vi "Send_Data.vi"(0 "Poss":dbl) -> (1 "value":dbl, 2 "error out":errorcluster)   [LabVIEW 2017]
uses:
  <vilib>/myRIO/Instrument Drivers/Onboard IO/AI Block/typedefs/AI Block Reference.ctl
  <vilib>/myRIO/Common/Instrument Driver Framework/Utilities/typedefs/myRIO Generic Hardware Reference.ctl
  <vilib>/myRIO/Common/Instrument Driver Framework/Utilities/typedefs/Hardware Version Enum.ctl
  <vilib>/myRIO/Common/Instrument Driver Framework/Utilities/typedefs/myRIO v1.0 Reference.ctl
  <vilib>/myRIO/Common/Instrument Driver Framework/Utilities/typedefs/Generic FPGA Reference.ctl
  <vilib>/myRIO/Common/Instrument Driver Framework/myRIO v1.0/AI Block/typedefs/AI Block Channels List.ctl
  <vilib>/myRIO/Common/Instrument Driver Framework/myRIO v1.0/AI Block/typedefs/AI Block Channels Enum.ctl
  <vilib>/myRIO/Common/Instrument Driver Framework/Utilities/typedefs/Analog Scaling Constants.ctl
  <vilib>/userdefined/High Color/nirio_resource_hc.ctl
  <vilib>/myRIO/Common/Instrument Driver Framework/Utilities/vis/Is FPGA Ref Available.vi
  <vilib>/myRIO/Common/Instrument Driver Framework/myRIO v1.0/AI Block/vis/myRIO v1.1 Open Throughput AI (N Samples).vi
  <vilib>/myRIO/Instrument Drivers/Onboard IO/AI Block/vis/Read.vi
  <vilib>/myRIO/Common/Instrument Driver Framework/Utilities/vis/Validate Channels.vi
  <vilib>/Utility/VariantDataType/GetNumericInfo.vi
  <vilib>/Utility/error.llb/Error Cluster From Error Code.vi
  <vilib>/myRIO/Common/Instrument Driver Framework/myRIO v1.0/myRIO v1.1 Open Throughput.vi
  <vilib>/myRIO/Common/Instrument Driver Framework/myRIO v1.0/AI Block/vis/myRIO v1.0 Get Scaling Constants AI Block.vi
  <vilib>/myRIO/Common/Instrument Driver Framework/myRIO v1.0/AI Block/vis/myRIO v1.0 Reserve AI Block.vi
  <vilib>/myRIO/Common/Instrument Driver Framework/myRIO v1.0/myRIO v1.0 Close.vi
  <vilib>/myRIO/Common/Instrument Driver Framework/myRIO v1.0/AI Block/vis/myRIO v1.0 AI Block Read.vi
  <vilib>/myRIO/Express VI/Onboard IO/AI/AI Express VI.xnode
  <vilib>/myRIO/Instrument Drivers/Onboard IO/AI Block/vis/myRIO AI N Samples Open.xnode
  <vilib>/myRIO/Instrument Drivers/Onboard IO/AI Block/AI Block.lvlib
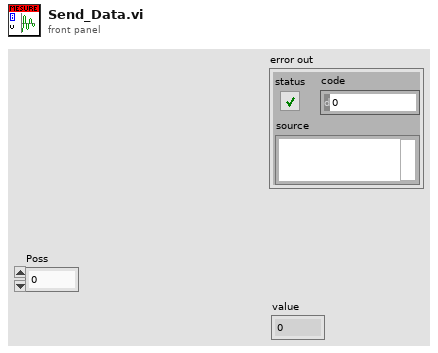
[diagram p1: front panel]
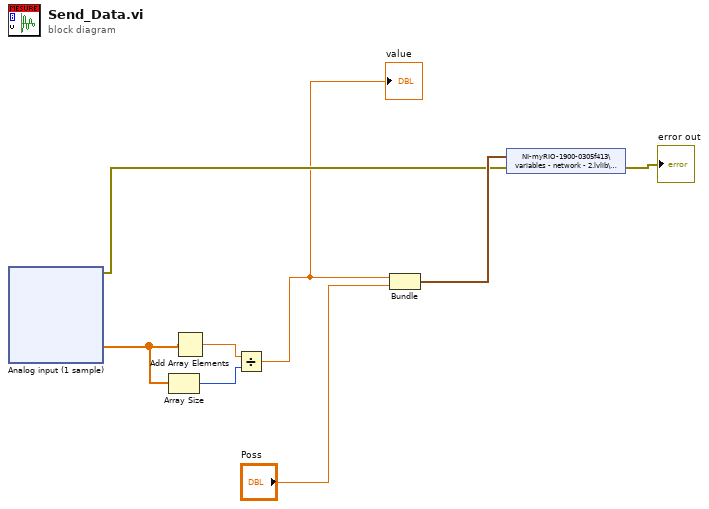
[diagram p0: block diagram]
diagram:
  n1 = xnode "Analog input (1 sample)"() -> ("A/AI0 (N Samples) (Pin 3)"=w4:dbl[], "error out"=w5:errorcluster)  [unwired: 1 in]
  n2 = Array Size(array=w4) -> (size(s)=w2:i32)
  n3 = Add Array Elements(numeric array=w4) -> (sum=w3:dbl)
  n4 = Divide(x=w3, y=w2) -> (x/y=w1:dbl)
  "value" <- w1
  n5 = Bundle(w1, "Poss"="Poss") -> (w6:cluster{dbl, "Poss":dbl})  [unwired: 1 in]
  n6 = shared-variable "NI-myRIO-1900-0305f413\\variables - network - 2.lvlib\\output cluster"(w6, error in=w5) -> (error out=→"error out":errorcluster)
